vi "MX100 Get Data.vi"(0 "VISA Refnum in":refnum<visa-resource-name>, 7 "MX100 Cluster In":T2={"Base Time"=0, "Session Number"=0, "Last Data Number"={"High"=-1, "Low"=4294967295}, "Channel List"=[], "FIFO Number (0)"=0, "Channel Number (1)"=1, "Select FIFO or Channel (F:Channel)"=FALSE, "MX100 Data"={"Measurement Values out"=[], "Date/Time"=""}} {"Channel Number (1)" min=1 max=60 step=1; "FIFO Number (0)" min=-1 max=2 step=1}, 11 "error in (no error)":errorcluster) -> (4 "VISA Refnum out":refnum<visa-resource-name>, 6 "Measurement Date Times":T1(array[cluster]), 8 "MX100 Cluster Out":T2={"Base Time"=0, "Session Number"=0, "Last Data Number"={"High"=-1, "Low"=4294967295}, "Channel List"=[], "FIFO Number (0)"=0, "Channel Number (1)"=1, "Select FIFO or Channel (F:Channel)"=FALSE, "MX100 Data"={"Measurement Values out"=[], "Date/Time"=""}} {"Channel Number (1)" min=1 max=60 step=1; "FIFO Number (0)" min=-1 max=2 step=1}, 10 "Measurement Values":dbl[][](array[numeric]), 15 "error out":errorcluster)   [LabVIEW 2016]
uses:
  Type Definitions/MX100 Initialization.ctl
  Type Definitions/MX100 Data.ctl
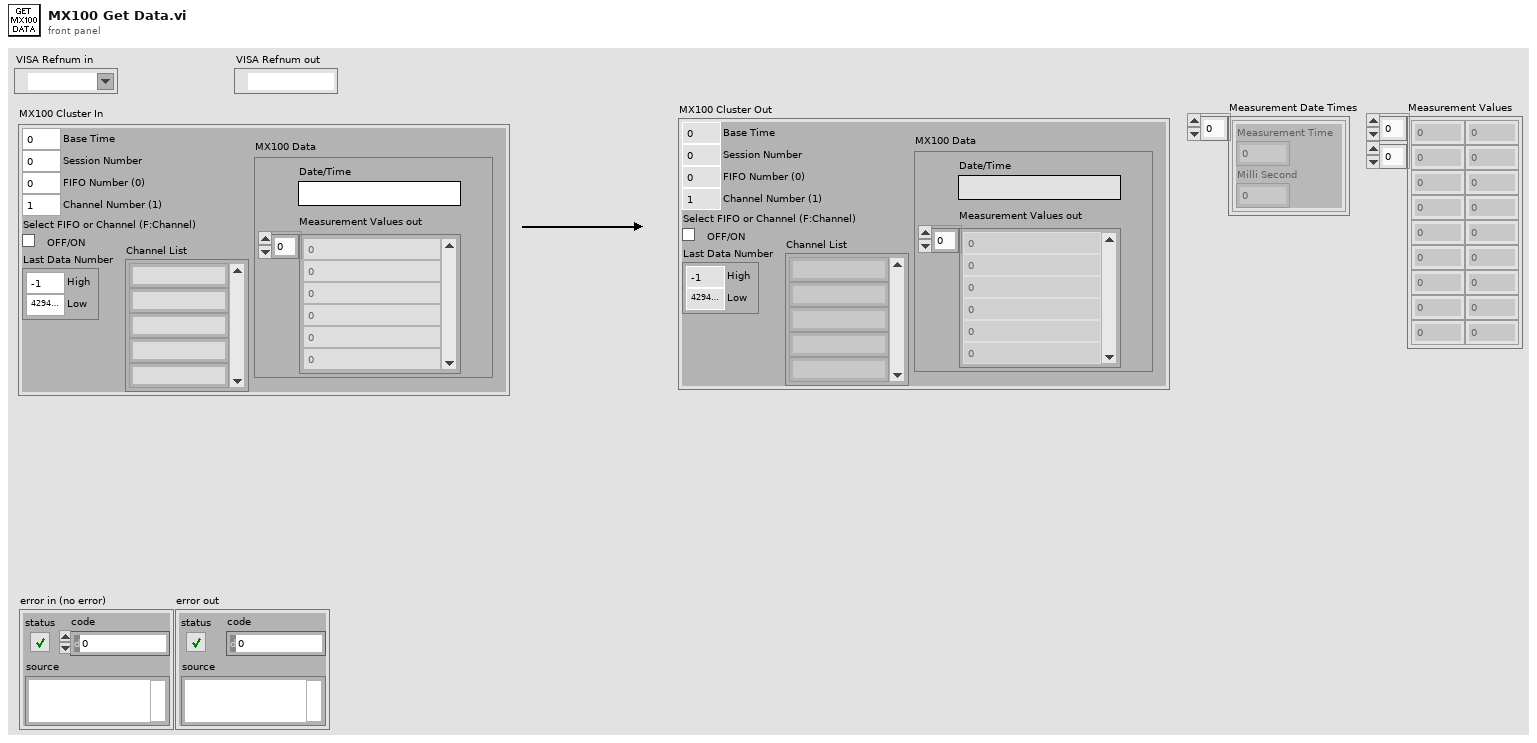
[diagram p1: front panel]
types:
  T1 = cluster{"Measurement Time":u32, "Milli Second":i32}[]
  T2 = typedef "MX100 Initialization.ctl" = cluster{"Base Time":i32, "Session Number":i32, "Last Data Number":cluster{"High":i32, "Low":u32}, "Channel List":string[], "FIFO Number (0)":i32, "Channel Number (1)":i32, "Select FIFO or Channel (F:Channel)":bool, "MX100 Data":T3}
  T3 = typedef "MX100 Data.ctl" = cluster{"Measurement Values out":dbl[], "Date/Time":string}
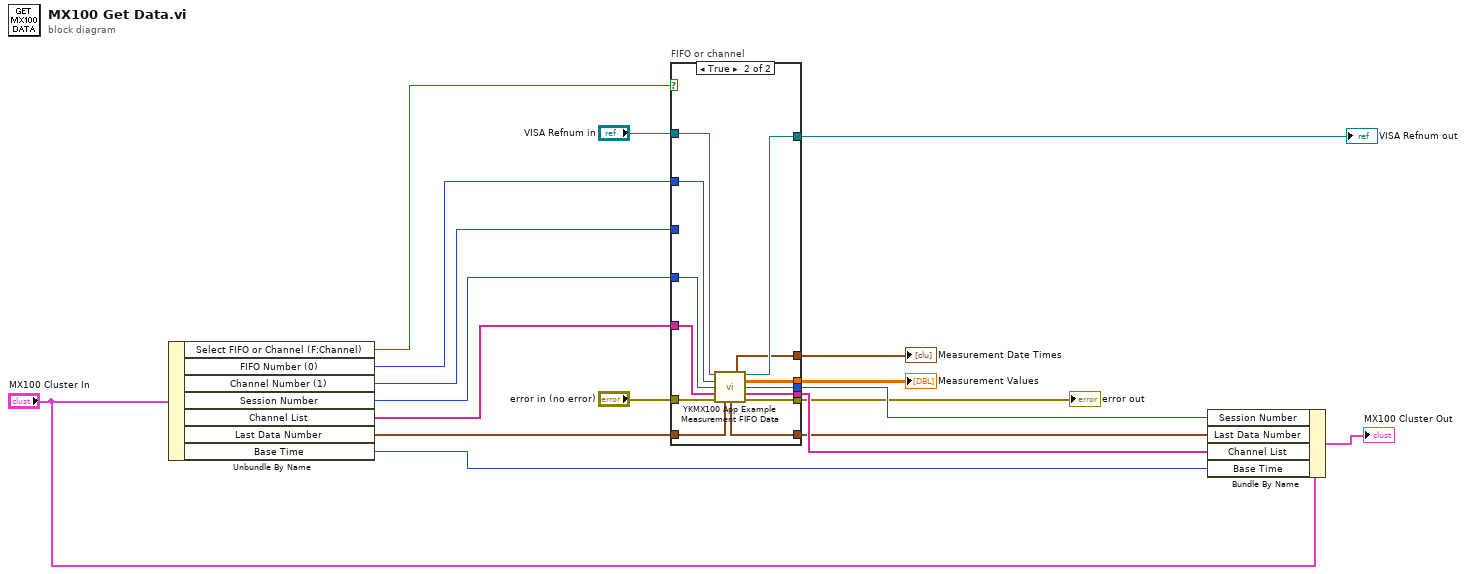
[diagram p0: block diagram]
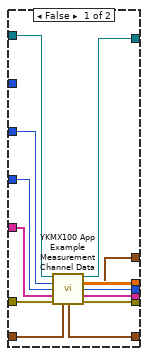
[diagram p2: hidden frame]
diagram:
  n1 = Unbundle By Name("MX100 Cluster In") -> ("Select FIFO or Channel (F:Channel)"=w6:bool, "FIFO Number (0)"=w8:i32, "Channel Number (1)"=w7:i32, "Session Number"=w14:i32, "Channel List"=w15:string[], "Last Data Number"=w13:cluster{"High":i32, "Low":u32}, "Base Time"=w4:i32)
  n2 = case "FIFO or channel" shown="True" w6 {
    tunnel: "VISA Refnum in" -> [w31 w44]
    tunnel: "error in (no error)" -> [w30 w43]
    tunnel: w8 -> [_ w42]
    tunnel: w7 -> [w29 _]
    tunnel: [w27 w41] -> w1
    tunnel: [w28 w40] -> w18
    tunnel: w15 -> [w26 w39]
    tunnel: [w25 w38] -> w11
    tunnel: w13 -> [w24 w37]
    tunnel: [w19 w32] -> w10
    tunnel: [w23 w36] -> w2
    tunnel: w14 -> [w22 w35]
    tunnel: [w21 w34] -> w5
    tunnel: [w20 w33] -> w3
    frame False {
      n3 = call "YKMX100 App Example Measurement Channel Data.vi"("VISA session"=w31, "Channel Number (1)"=w29, "Session Number (-1)"=w22, "Channel Info List (no array)"=w26, "error in (no error)"=w30, "Last Data Number (-1)"=w24) -> ("Measurement Date Times"=w20:T1, "dup VISA session"=w28:refnum<visa-resource-name>, "Measurement Values"=w23:dbl[][], "Session Number"=w21:i32, "Channel Info List"=w25:string[], "End Data Number"=w19:cluster{"High":i32, "Low":u32}, "error out"=w27:errorcluster)  [unwired: 2 in, 1 out]
    }
    frame True {
      n4 = call "YKMX100 App Example Measurement FIFO Data.vi"("VISA session"=w44, "FIFO Number (0)"=w42, "Session Number (-1)"=w35, "Channel Info List (no array)"=w39, "error in (no error)"=w43, "Last Data Number (-1)"=w37) -> ("Measurement Date Times"=w33:T1, "dup VISA session"=w40:refnum<visa-resource-name>, "Measurement Values"=w36:dbl[][], "Session Number"=w34:i32, "Channel Info List"=w38:string[], "End Data Number"=w32:cluster{"High":i32, "Low":u32}, "error out"=w41:errorcluster)  [unwired: 2 in, 1 out]
    }
  }
  "error out" <- w1
  "VISA Refnum out" <- w18
  "Measurement Date Times" <- w3
  "Measurement Values" <- w2
  n5 = Bundle By Name(cluster="MX100 Cluster In", "Session Number"=w5, "Last Data Number"=w10, "Channel List"=w11, "Base Time"=w4) -> (→"MX100 Cluster Out":T2)
